vi "cost.vi"(8 "error in (no error)":errorcluster, 11 "Mocha in":refnum<class "Mocha.lvclass">) -> (0 "error out":errorcluster, 2 "Cost":dbl, 3 "Mocha out":refnum<class "Mocha.lvclass">)   [LabVIEW 2013, in "Mocha.lvclass"]
uses:
  Mocha.lvclass
  Mocha.lvclass/Mocha.ctl
  Beverage/Beverage.lvclass
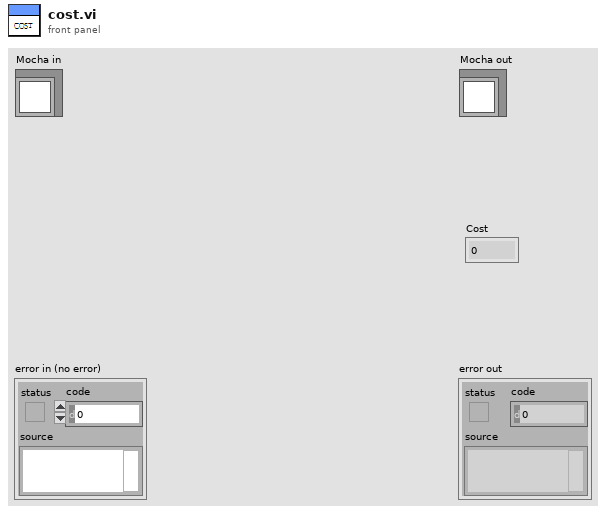
[diagram p1: front panel]
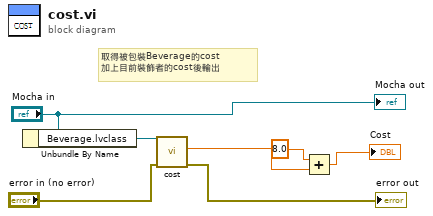
[diagram p0: block diagram]
diagram:
  # "取得被包裝Beverage的cost\n加上目前裝飾者的cost後輸出"
  n1 = Unbundle By Name("Mocha in") -> ("Beverage.lvclass"=w5:refnum<class "Beverage.lvclass">)
  n2 = call-dynamic "cost.vi"("error in (no error)"="error in (no error)", "Beverage in"=w5) -> ("error out"=→"error out":errorcluster, "Cost"=w2:dbl)  [unwired: 7 in, 1 out]
  n3 = Add(x=8.0 ("Cost"), y=w2) -> (x+y=→"Cost":dbl)
  "Mocha out" <- "Mocha in"
